vi "test-linear-system-id.vi"() -> ()   [LabVIEW 2019]
uses:
  <vilib>/Rock Robotics/WPI/ThirdParty/JAS_Junk/TrajLib/LINEAR_SYSTEM.ctl
  <vilib>/Analysis/Matrix/Datatypes/RealMatrix.ctl
  <vilib>/Rock Robotics/WPI/ThirdParty/JAS_Junk/TrajLib/LinearSystem_New.vi
  <vilib>/Rock Robotics/WPI/ThirdParty/JAS_Junk/TrajLib/MatBuilder_Create.vi
  <vilib>/Rock Robotics/WPI/ThirdParty/JAS_Junk/TrajLib/MatrixHelper_Zero.vi
  <vilib>/Rock Robotics/WPI/ThirdParty/JAS_Junk/TrajLib/MatBuilder_Fill.vi
  <vilib>/Rock Robotics/WPI/ThirdParty/JAS_Junk/TrajLib/DCMotor_New.vi
  <vilib>/Rock Robotics/WPI/ThirdParty/JAS_Junk/TrajLib/Units_RotationsPerMinuteToRadiansPerSecond.vi
  <vilib>/Rock Robotics/WPI/ThirdParty/JAS_Junk/TrajLib/MatrixHelper_CoerceSize.vi
  <vilib>/Analysis/7linalg.llb/Create Special Matrix.vi
  <vilib>/Analysis/7linalg.llb/Create Special Real Matrix.vi
  <vilib>/Rock Robotics/WPI/ThirdParty/JAS_Junk/TrajLib/Trajectory_Library.lvlib
  <vilib>/Analysis/Matrix/NI_Matrix.lvlib
panel:
  out "IdentifyVelocitySystem":T1
  out "IdentifyPositionSystem":T1
  out "FlyWheel":T1
  out "DriveTrain":T1
  out "Elevator":T1
  # "A  = -10.14132, 3.06598, \n            3.06598, -10.14132\n\nB =    4.2590,   -1.28762, \n         -1.2876,   4.2590\n\nC =   1.0,   0.0, \n          0.0,  1.0;\n\nD =   0.0,   0.0, \n          0.0,   0.0"
  # "A   = (0, 1, \n               0, -99.05473)\n\n     B = (0, \n            20.8)\n\n   C   = 1, 0\n\n    D = 0"
  # "A = -26.87032\n\nB = 1354.166667;\n\nC = 1\n\nD = 0"
  # "A =   0, 1, \n         0, -1 / 0.5\n\nB =  0, \n        1 / 0.5"
  # "A =   -1.0 / 0.5\n\nB = 1 / 0.5"
  # "<States,States>"
  # "<States,Inputs>"
  # "<Outputs,States>"
  # "<Outputs,Inputs>"
  # "<States,States>"
  # "<States,Inputs>"
  # "<Outputs,States>"
  # "<Outputs,Inputs>"
  # "<States,States>"
  # "<States,Inputs>"
  # "<Outputs,States>"
  # "<Outputs,Inputs>"
  # "<States,States>"
  # "<States,Inputs>"
  # "<Outputs,States>"
  # "<Outputs,Inputs>"
  # "<States,States>"
  # "<States,Inputs>"
  # "<Outputs,States>"
  # "<Outputs,Inputs>"
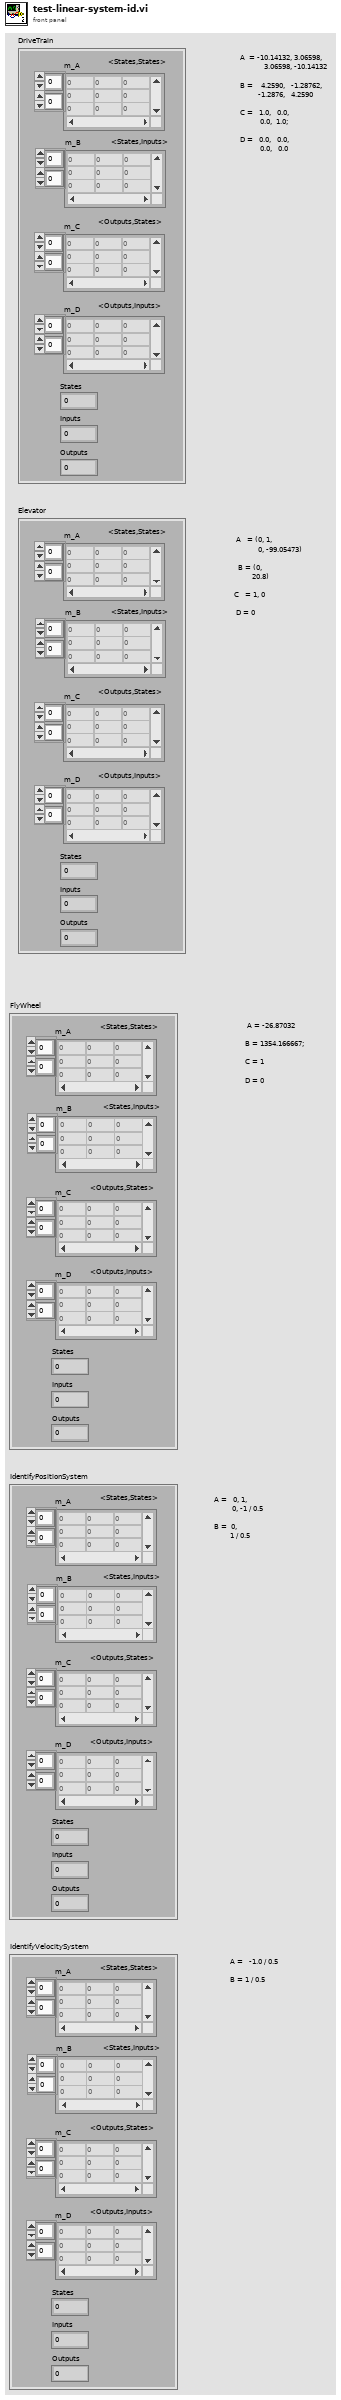
[diagram p1: front panel]
types:
  T1 = typedef "Trajectory_Library.lvlib/LINEAR_SYSTEM.ctl" = cluster{"m_A":T2, "m_B":T2, "m_C":T2, "m_D":T2, "States":i32, "Inputs":i32, "Outputs":i32}
  T2 = typedef "NI_Matrix.lvlib/RealMatrix.ctl" = dbl[][]
  T3 = typedef "Trajectory_Library.lvlib/DCMOTOR.CTL" = cluster{"nominalVoltage_Volts":dbl, "StallTorque_NM":dbl, "StallCurrent_Amps":dbl, "FreeCurrent_Amps":dbl, "FreeSpeed_RadPerSec":dbl, "R_Ohms":dbl, "Kv_RadPerSecPerVolt":dbl, "Kt_NMPerAmp":dbl}
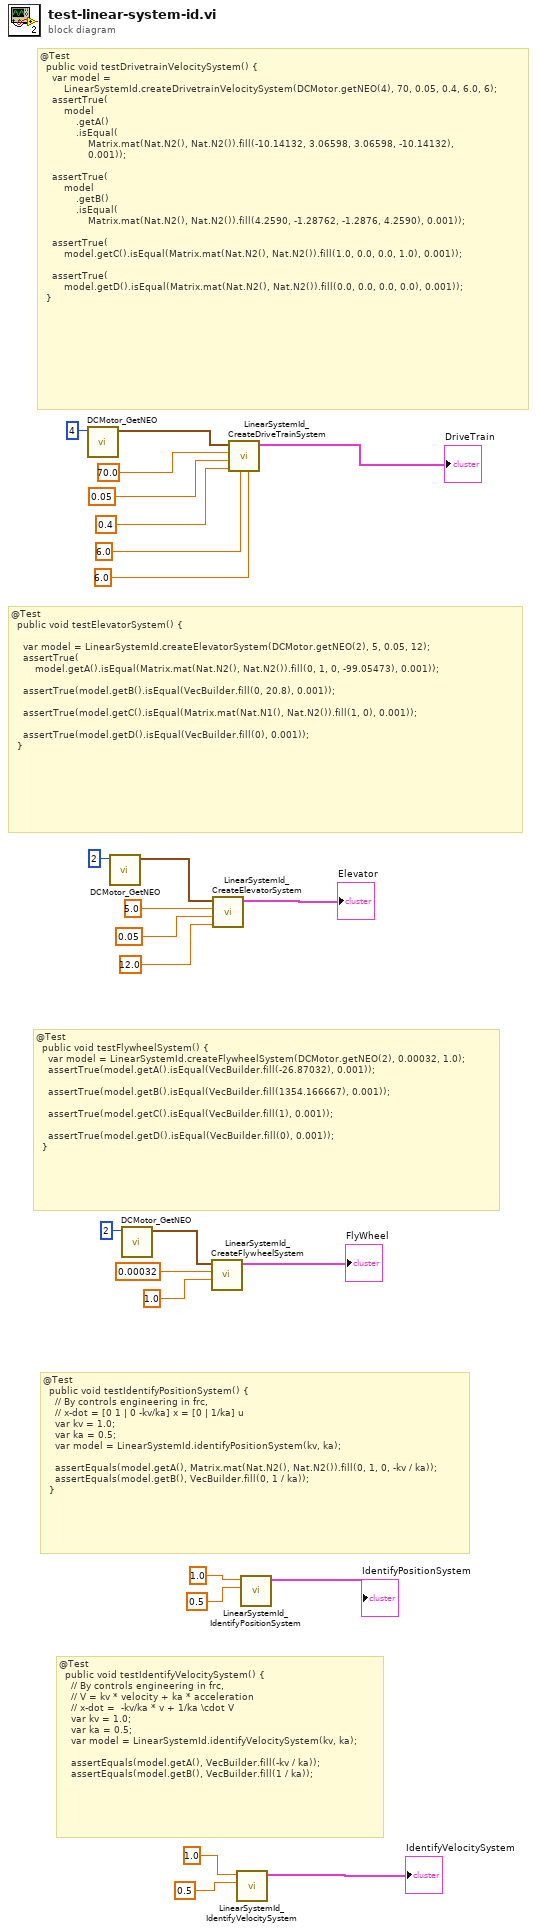
[diagram p0: block diagram]
diagram:
  # "@Test\n  public void testIdentifyVelocitySystem() {\n    // By controls engineering in frc,\n    // V = kv * velocity + ka * acceleration\n    // x-dot =  -kv/ka * v + 1/ka \\cdot V\n    var kv = 1.0;\n    var ka = 0.5;\n    var model = LinearSystemId.identifyVelocitySystem(kv, ka);\n\n    assertEquals(model.getA(), VecBuilder.fill(-kv / ka));\n    assertEquals(model.getB(), VecBuilder.fill(1 / ka));"
  # "@Test\n  public void testIdentifyPositionSystem() {\n    // By controls engineering in frc,\n    // x-dot = [0 1 | 0 -kv/ka] x = [0 | 1/ka] u\n    var kv = 1.0;\n    var ka = 0.5;\n    var model = LinearSystemId.identifyPositionSystem(kv, ka);\n\n    assertEquals(model.getA(), Matrix.mat(Nat.N2(), Nat.N2()).fill(0, 1, 0, -kv / ka));\n    assertEquals(model.getB(), VecBuilder.fill(0, 1 / ka));\n  }"
  # "@Test\n  public void testFlywheelSystem() {\n    var model = LinearSystemId.createFlywheelSystem(DCMotor.getNEO(2), 0.00032, 1.0);\n    assertTrue(model.getA().isEqual(VecBuilder.fill(-26.87032), 0.001));\n\n    assertTrue(model.getB().isEqual(VecBuilder.fill(1354.166667), 0.001));\n\n    assertTrue(model.getC().isEqual(VecBuilder.fill(1), 0.001));\n\n    assertTrue(model.getD().isEqual(VecBuilder.fill(0), 0.001));\n  }"
  # "@Test\n  public void testDrivetrainVelocitySystem() {\n    var model =\n        LinearSystemId.createDrivetrainVelocitySystem(DCMotor.getNEO(4), 70, 0.05, 0.4, 6.0, 6);\n    assertTrue(\n        model\n            .getA()\n            .isEqual(\n                Matrix.mat(Nat.N2(), Nat.N2()).fill(-10.14132, 3.06598, 3.06598, -10.14132),\n                0.001));\n\n    assertTrue(\n        model\n            .getB()\n            .isEqual(\n                Matrix.mat(Nat.N2(), Nat.N2()).fill(4.2590, -1.28762, -1.2876, 4.2590), 0.001));\n\n    assertTrue(\n        model.getC().isEqual(Matrix.mat(Nat.N2(), Nat.N2()).fill(1.0, 0.0, 0.0, 1.0), 0.001));\n\n    assertTrue(\n        model.getD().isEqual(Matrix.mat(Nat.N2(), Nat.N2()).fill(0.0, 0.0, 0.0, 0.0), 0.001));\n  }"
  # "@Test\n  public void testElevatorSystem() {\n\n    var model = LinearSystemId.createElevatorSystem(DCMotor.getNEO(2), 5, 0.05, 12);\n    assertTrue(\n        model.getA().isEqual(Matrix.mat(Nat.N2(), Nat.N2()).fill(0, 1, 0, -99.05473), 0.001));\n\n    assertTrue(model.getB().isEqual(VecBuilder.fill(0, 20.8), 0.001));\n\n    assertTrue(model.getC().isEqual(Matrix.mat(Nat.N1(), Nat.N2()).fill(1, 0), 0.001));\n\n    assertTrue(model.getD().isEqual(VecBuilder.fill(0), 0.001));\n  }"
  n1 = call <vilib>:"DCMotor_GetNEO.vi"("Num Motors"=4) -> ("DCMOTOR"=w18:T3)  [unwired: 10 in]
  n2 = call <vilib>:"DCMotor_GetNEO.vi"("Num Motors"=2) -> ("DCMOTOR"=w24:T3)  [unwired: 10 in]
  n3 = call <vilib>:"DCMotor_GetNEO.vi"("Num Motors"=2) -> ("DCMOTOR"=w10:T3)  [unwired: 10 in]
  n4 = call <vilib>:"LinearSystemId_CreateFlywheelSystem.vi"("G"=1.0, "jKgMetersSquared"=0.00032, "DCMOTOR"=w10) -> ("Linearsystem"=→"FlyWheel":T1)  [unwired: 8 in]
  n5 = call <vilib>:"LinearSystemId_CreateElevatorSystem.vi"("G"=12.0, "radiusMeters"=0.05, "massKg"=5.0, "DCMOTOR"=w24) -> ("Linearsystem"=→"Elevator":T1)  [unwired: 7 in]
  n6 = call <vilib>:"LinearSystemId_CreateDriveTrainSystem.vi"("G"=6.0, "JKgMetersSquared"=6.0, "rbMeters"=0.4, "rMeters"=0.05, "MassKg"=70.0, "Motor"=w18) -> ("Linearsystem"=→"DriveTrain":T1)  [unwired: 5 in]
  n7 = call <vilib>:"LinearSystemId_IdentifyVelocitySystem.vi"("kA"=0.5, "kV"=1.0) -> ("Linearsystem"=→"IdentifyVelocitySystem":T1)  [unwired: 9 in]
  n8 = call <vilib>:"LinearSystemId_IdentifyPositionSystem.vi"("kA"=0.5, "kV"=1.0) -> ("Linearsystem"=→"IdentifyPositionSystem":T1)  [unwired: 9 in]
